vi "ColorWheelSystem.vi"(8 "Manual spin":dbl, 11 "SecondaryJoystickButtons":T1) -> ()   [LabVIEW 2019]
uses:
  Controls/SecondaryJoystickButtons.ctl
panel:
  # "Z Axis goes in the open terminal"
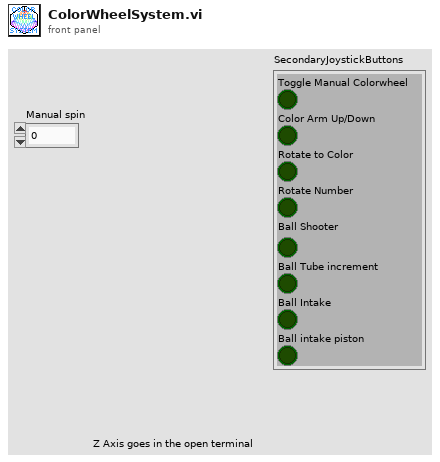
[diagram p1: front panel]
types:
  T1 = typedef "SecondaryJoystickButtons.ctl" = cluster{"Toggle Manual Colorwheel":bool, "Color Arm Up/Down":bool, "Rotate to Color":bool, "Rotate Number":bool, "Ball Shooter":bool, "Ball Tube increment":bool, "Ball Intake":bool, "Ball intake piston":bool}
  T2 = typedef "WPI_SolenoidValue.ctl" = enum16{"Off", "On", "Forward", "Reverse"}
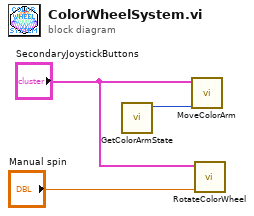
[diagram p0: block diagram]
diagram:
  n1 = call "GetColorArmState.vi"() -> ("Arm Valve State"=w1:T2)  [unwired: 11 in]
  n2 = call "MoveColorArm.vi"("Arm Valve State"=w1, "SecondaryJoystickButtons"="SecondaryJoystickButtons") -> ()  [unwired: 10 in]
  n3 = call "RotateColorWheel.vi"("Manual Spin"="Manual spin", "SecondaryJoystickButtons"="SecondaryJoystickButtons") -> ()  [unwired: 10 in]
